vi "Contrast.vi"(1 "Y2":dbl, 2 "Y1":dbl) -> (0 "(max(Y1,Y2) - min(Y1,Y2)) / (Y1 + Y2)":dbl)   [LabVIEW 2019]
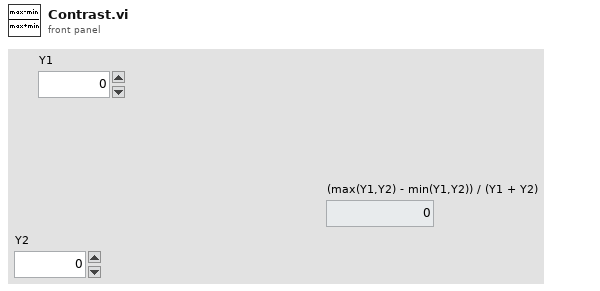
[diagram p1: front panel]
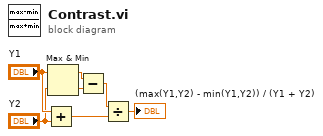
[diagram p0: block diagram]
diagram:
  n1 = Add(x="Y1", y="Y2") -> (x+y=w2:dbl)
  n2 = Max & Min(x="Y1", y="Y2") -> (max(x,y)=w7:dbl, min(x,y)=w6:dbl)
  n3 = Subtract(x=w7, y=w6) -> (x-y=w3:dbl)
  n4 = Divide(x=w3, y=w2) -> (x/y=→"(max(Y1,Y2) - min(Y1,Y2)) / (Y1 + Y2)":dbl)
